vi "Textformatter.vi"() -> ()   [LabVIEW 2015]
panel:
  out "Output":string
  in  "Select Operation":string(combo)
  in  "Input":string
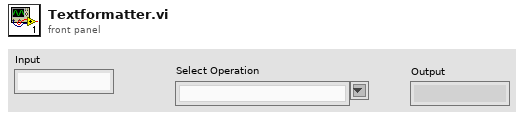
[diagram p1: front panel]
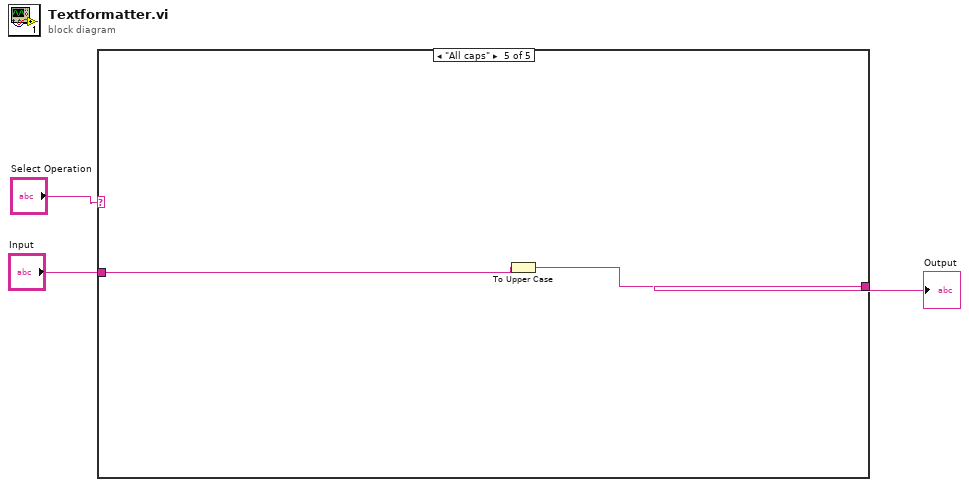
[diagram p0: block diagram]
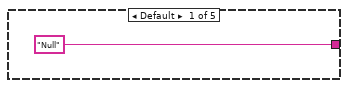
[diagram p2: hidden frame]
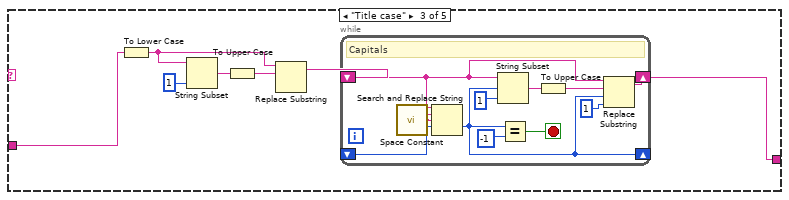
[diagram p4: hidden frame]
diagram:
  n1 = case shown="\"All caps\"" "Select Operation" {
    tunnel: ["Null" w5 w6 w24 w25] -> w3
    tunnel: "Input" -> [_ w5 w7 w24 w26]
    frame Default {
    }
    frame "Start Case" {
    }
    frame "Title case" {
      n2 = To Lower Case(string=w7) -> (all lower case string=w11:string)
      n3 = String Subset(string=w11, length (rest)=1 ("length (rest)")) -> (substring=w10:string)  [unwired: 1 in]
      n4 = To Upper Case(1:w10) -> (0:w9:string)
      n5 = Replace Substring(4:w9, 5:w11) -> (1:w8:string)  [unwired: 2 in, 1 out]
      n6 = while {
        shift-right: [w17] -> w6
        shift-left: w8 -> [w19]
        shift-right: [w15] -> _
        shift-left: _ -> [w16]
        stop <- w13 stop-if-true
        # "Capitals"
        n7 = call <vilib>:"Space Constant.vi"() -> ("String"=w23:string)
        n8 = Search and Replace String(input string=w19, search string=w23, replace string=w23, offset=w16) -> (offset past replacement=w15:i32)  [unwired: 4 in, 3 out]
        n9 = String Subset(string=w19, offset (0)=w15, length (rest)=1 ("length (rest)")) -> (substring=w21:string)
        n10 = Equal?(x=w15, y=-1) -> (x = y?=w13:bool)
        n11 = To Upper Case(1:w21) -> (0:w20:string)
        n12 = Replace Substring(2:1 ("length (len. of substring)"), 3:w15, 4:w20, 5:w19) -> (1:w17:string)  [unwired: 1 out]
      }
    }
    frame "Small" {
    }
    frame "All caps" {
      n13 = To Upper Case(1:w26) -> (0:w25:string)
    }
  }
  "Output" <- w3
